vi "freq_scan_FRXYP.vi"() -> ()   [LabVIEW 2010]
uses:
  <vilib>/Utility/file.llb/Write To Spreadsheet File (DBL).vi
panel:
  in  "Path":path
  out "Waveform Chart":cluster{dbl, dbl}(graph)={-0.00102235, 0.00816351}
  out "amp":string="0.00823218"
  out "freq":string="2739.2"
  out "Amp vs Freq":cluster{dbl, dbl}[](graph)=[{2737.3999999999987, 0.036278}, {2737.5999999999985, 0.0290834}, {2737.7999999999984, 0.0244981}, {2736.0, 0.00607303}, {2736.2, 0.0105897}, {2736.3999999999996, 0.0156404}, {2736.5999999999995, 0.0193788}, {2736.7999999999993, 0.0272676}, {2736.999999999999, 0.0}, {2736.0, 0.0158159}, {2736.2, 0.014473}, {2736.3999999999996, 0.0187455}, {2736.5999999999995, 0.0252458}, {2736.7999999999993, 0.035187}, {2736.999999999999, 0.0429919}, {2737.199999999999, 0.0378878}, {2737.3999999999987, 0.0261461}, {2737.5999999999985, 0.0193864}, {2736.0, 0.00734714}, {2736.2, 0.0133744}, {2736.3999999999996, 0.0180436}, {2736.5999999999995, 0.0241624}, {2736.7999999999993, 0.0333941}, {2736.999999999999, 0.042145}, {2737.199999999999, 0.037575}, {2737.3999999999987, 0.0249025}, {2737.5999999999985, 0.0186692}, {2737.7999999999984, 0.014618}, {2737.999999999998, 0.0118027}, {2738.199999999998, 0.010666}, {2738.399999999998, 0.0110856}, {2738.5999999999976, 0.00988775}, {2738.7999999999975, 0.00891882}, {2738.9999999999973, 0.00823218}]
  in  "Driving amplitude (0 Vrms:0)":cluster{ext, i32}={0.2, 0} {"?" items=["Vrms", "Vpp", "dBm"]; "?" format="%.3f"}
  in  "Step interval in ms":u32=1500
  in  "Step in Hz":dbl=0.2 min=0.0 format="%.2f"
  in  "Unit":i8=1 min=0 max=2 step=1
  in  "End Frequency":dbl=2.743 min=0.0 format="%.3f"
  in  "Start Frequency":dbl=2.736 min=0.0 format="%.3f"
  in  "On/Off":bool=TRUE
  # "Make sure to set DS345's GPIB address to 19.\nMake sure to set SR830's GPIB address to 8."
  # "0: Hz\n1: kHz\n2: MHz"
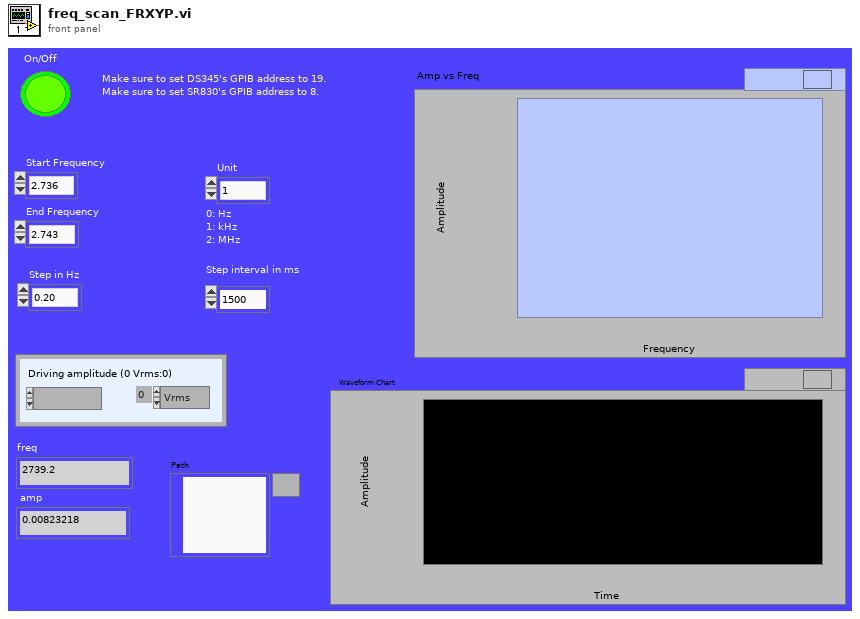
[diagram p1: front panel]
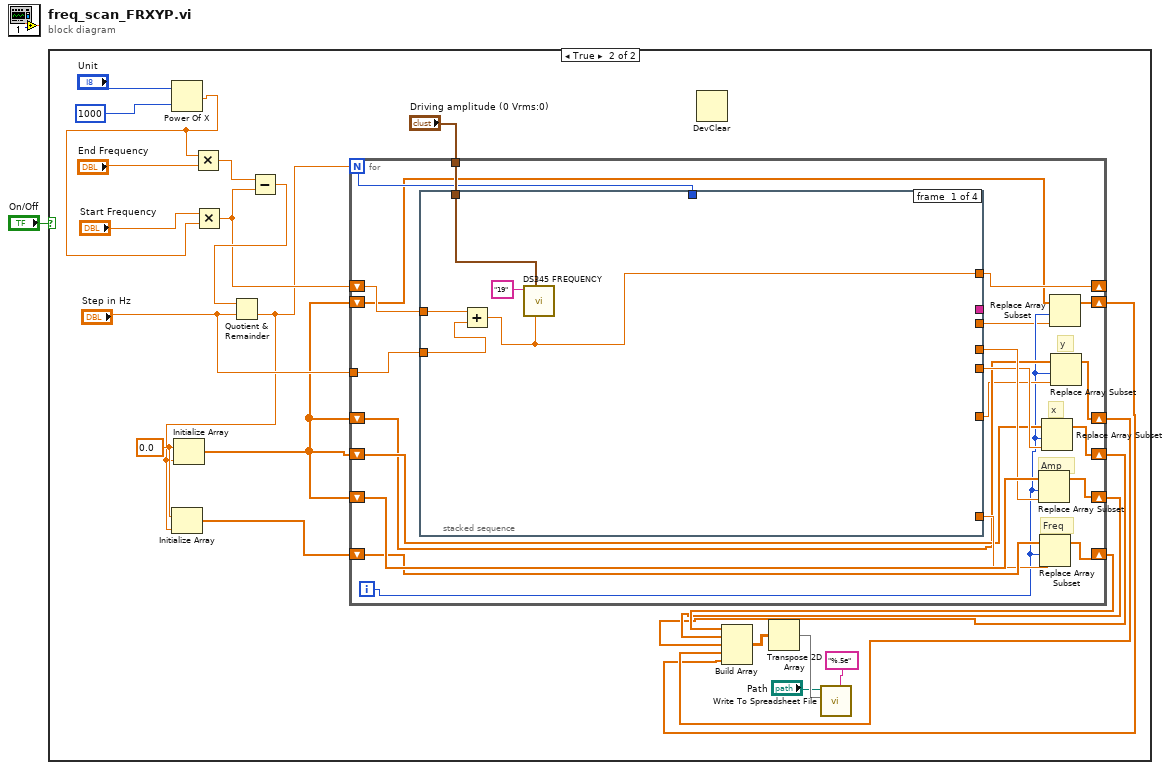
[diagram p0: block diagram]
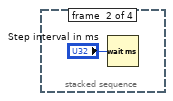
[diagram p3: hidden frame]
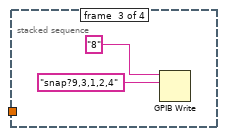
[diagram p4: hidden frame]
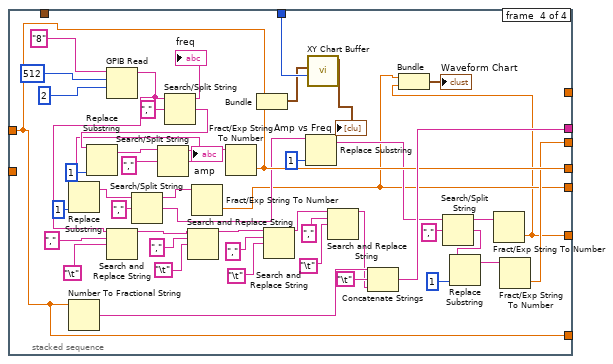
[diagram p5: hidden frame]
diagram:
  n1 = case shown="True" "On/Off" {
    frame False {
    }
    frame True {
      w14 = 0.0 ("element")
      n2 = Power Of X(1:1000, 2:"Unit") -> (0:w22:dbl)
      n3 = Multiply(x=w22, y="End Frequency") -> (x*y=w18:dbl)
      n4 = Multiply(x="Start Frequency", y=w22) -> (x*y=w17:dbl)
      n5 = Subtract(x=w18, y=w17) -> (x-y=w19:dbl)
      n6 = Quotient & Remainder(x=w19, y="Step in Hz") -> (floor(x/y)=w13:dbl)  [unwired: 1 out]
      n7 = Initialize Array(w14, w13) -> (w12:dbl[])
      n8 = Initialize Array(w14, w13) -> (w8:dbl[])
      n9 = for {
        N: w13 -> [w42]
        shift-right: [w29] -> _
        shift-left: w17 -> [w44]
        tunnel: "Step in Hz" -> [w45]
        tunnel: "Driving amplitude (0 Vrms:0)" -> [w43]
        shift-right: [w40] -> w5
        shift-left: w8 -> [w41]
        shift-right: [w37] -> w6
        shift-left: w12 -> [w39]
        shift-right: [w32] -> w4
        shift-left: w8 -> [w34]
        shift-right: [w30] -> w3
        shift-left: w8 -> [w33]
        shift-right: [w26] -> w2
        shift-left: w8 -> [w25]
        i -> [w28]
        # "Amp"
        # "Freq"
        # "x"
        # "y"
        n10 = stacked-sequence {
          tunnel: w45 -> [w48 _ _ _]
          tunnel: w44 -> [w50 _ _ w67]
          tunnel: [w49 _ _ _] -> w29
          tunnel: w43 -> [w46 _ _ _]
          tunnel: w42 -> [_ _ _ w96]
          tunnel: [_ _ _ w74] -> _
          tunnel: [_ _ _ w67] -> w38
          tunnel: [_ _ _ w72] -> w36
          tunnel: [_ _ _ w56] -> w35
          tunnel: [_ _ _ w55] -> w31
          tunnel: [_ _ _ w66] -> w27
          frame #0 {
            n11 = Add(x=w50, y=w48) -> (x+y=w49:dbl)
            n12 = call "DS345 FREQUENCY.vi"("GPIB address"="19", "amplitude (0 Vrms:0)"=w46, "frequency"=w49) -> ()  [unwired: 5 in, 1 out]
          }
          frame #1 {
            n13 = Wait (ms)(milliseconds to wait="Step interval in ms") -> ()  [unwired: 1 out]
          }
          frame #2 {
            n14 = GPIB Write(0:"8" ("address string"), 1:"snap?9,3,1,2,4" ("data")) -> ()  [unwired: 1 in, 4 out]
          }
          frame #3 {
            n15 = Number To Fractional String(number=w67) -> (F-format string=w76:string)  [unwired: 3 out]
            n16 = GPIB Read(0:"8" ("address string"), 1:512 ("byte count"), 2:i16 2 ("mode (0)")) -> (5:w88:string)  [unwired: 1 in, 3 out]
            n17 = Search and Replace String(input string=w88, search string=",", replace string="\t") -> (result string=w85:string)  [unwired: 1 in, 7 out]
            n18 = Search/Split String(string=w88, search string/char (-)=",") -> (substring before match=→"freq":string, match + rest of string=w93:string)  [unwired: 2 out]
            n19 = Replace Substring(2:1 ("length (len. of substring)"), 5:w93) -> (1:w91:string)  [unwired: 3 out]
            n20 = Search/Split String(string=w91, search string/char (-)=",") -> (substring before match=w89:string, match + rest of string=w64:string)  [unwired: 2 out]
            "amp" <- w89
            n21 = Replace Substring(2:1, 5:w64) -> (1:w63:string)  [unwired: 3 out]
            n22 = Search/Split String(string=w63, search string/char (-)=",") -> (substring before match=w70:string, match + rest of string=w61:string)  [unwired: 2 out]
            n23 = Search and Replace String(input string=w85, search string=",", replace string="\t") -> (result string=w82:string)  [unwired: 1 in, 7 out]
            n24 = Fract/Exp String To Number(string=w70) -> (number=w56:dbl)  [unwired: 4 out]
            n25 = Fract/Exp String To Number(string=w89) -> (number=w72:dbl)  [unwired: 4 out]
            n26 = Bundle(w67, w72) -> (w95:cluster{dbl, dbl})  [unwired: 1 out]
            n27 = Search and Replace String(input string=w82, search string=",", replace string="\t") -> (result string=w79:string)  [unwired: 1 in, 7 out]
            n28 = Replace Substring(2:1, 5:w61) -> (1:w60:string)  [unwired: 3 out]
            n29 = call "XY Chart Buffer.vi"("chart length (points)"=w96, "new point"=w95) -> ("XY chart data"=→"Amp vs Freq":cluster{"x":dbl, "y":dbl}[])  [unwired: 2 in, 7 out]
            n30 = Search and Replace String(input string=w79, search string=",", replace string="\t") -> (result string=w73:string)  [unwired: 1 in, 7 out]
            n31 = Concatenate Strings(w76, "\t", w73) -> (w74:string)
            n32 = Search/Split String(string=w60, search string/char (-)=",") -> (substring before match=w68:string, match + rest of string=w59:string)  [unwired: 2 out]
            n33 = Replace Substring(2:1, 5:w59) -> (1:w57:string)  [unwired: 3 out]
            n34 = Fract/Exp String To Number(string=w68) -> (number=w55:dbl)  [unwired: 4 out]
            n35 = Bundle(w56, w55) -> (→"Waveform Chart":cluster{dbl, dbl})  [unwired: 1 out]
            n36 = Fract/Exp String To Number(string=w57) -> (number=w66:dbl)  [unwired: 4 out]
          }
        }
        n37 = Replace Array Subset(array=w41, new element=w36, index=w28) -> (w40:dbl[])
        n38 = Replace Array Subset(array=w39, new element=w38, index=w28) -> (w37:dbl[])
        n39 = Replace Array Subset(array=w34, new element=w35, index=w28) -> (w32:dbl[])
        n40 = Replace Array Subset(array=w25, new element=w27, index=w28) -> (w26:dbl[])
        n41 = Replace Array Subset(array=w33, new element=w31, index=w28) -> (w30:dbl[])
      }
      n42 = DevClear() -> ()  [unwired: 1 in, 4 out]
      n43 = Build Array(w6, w5, w4, w3, w2) -> (w10:dbl[][])
      n44 = Transpose 2D Array(2D array=w10) -> (transposed array=w9:dbl[][])
      n45 = call-poly <vilib>:"Write To Spreadsheet File.vi"("format (%.3f)"="%.5e", "2D data"=w9, "file path (dialog if empty)"="Path") -> ()  [unwired: 3 in, 3 out]
    }
  }
